vi "Get or Add Style Index.vi"(8 "error in":errorcluster, 10 "Format":string="dd/mm/yy hh:mm:ss.000", 11 "SpreadsheetDocument in":refnum<k24>) -> (0 "error out":errorcluster, 2 "Style Index":u32, 3 "SpreadsheetDocument out":refnum<k24>)   [LabVIEW 2021, in "Open Xml.lvlib"]
uses:
  Open Xml.lvlib
  D:/git/Open-Xml-LabVIEW/dll/DocumentFormat.OpenXml.dll
  dll/DocumentFormat.OpenXml.dll
  D:/git/Open-Xml-LabVIEW/dll/DocumentFormat.OpenXml.Framework.dll
  dll/DocumentFormat.OpenXml.Framework.dll
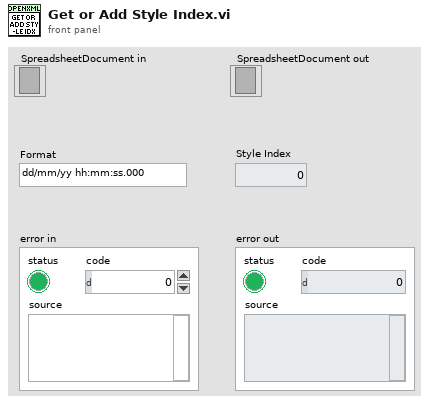
[diagram p1: front panel]
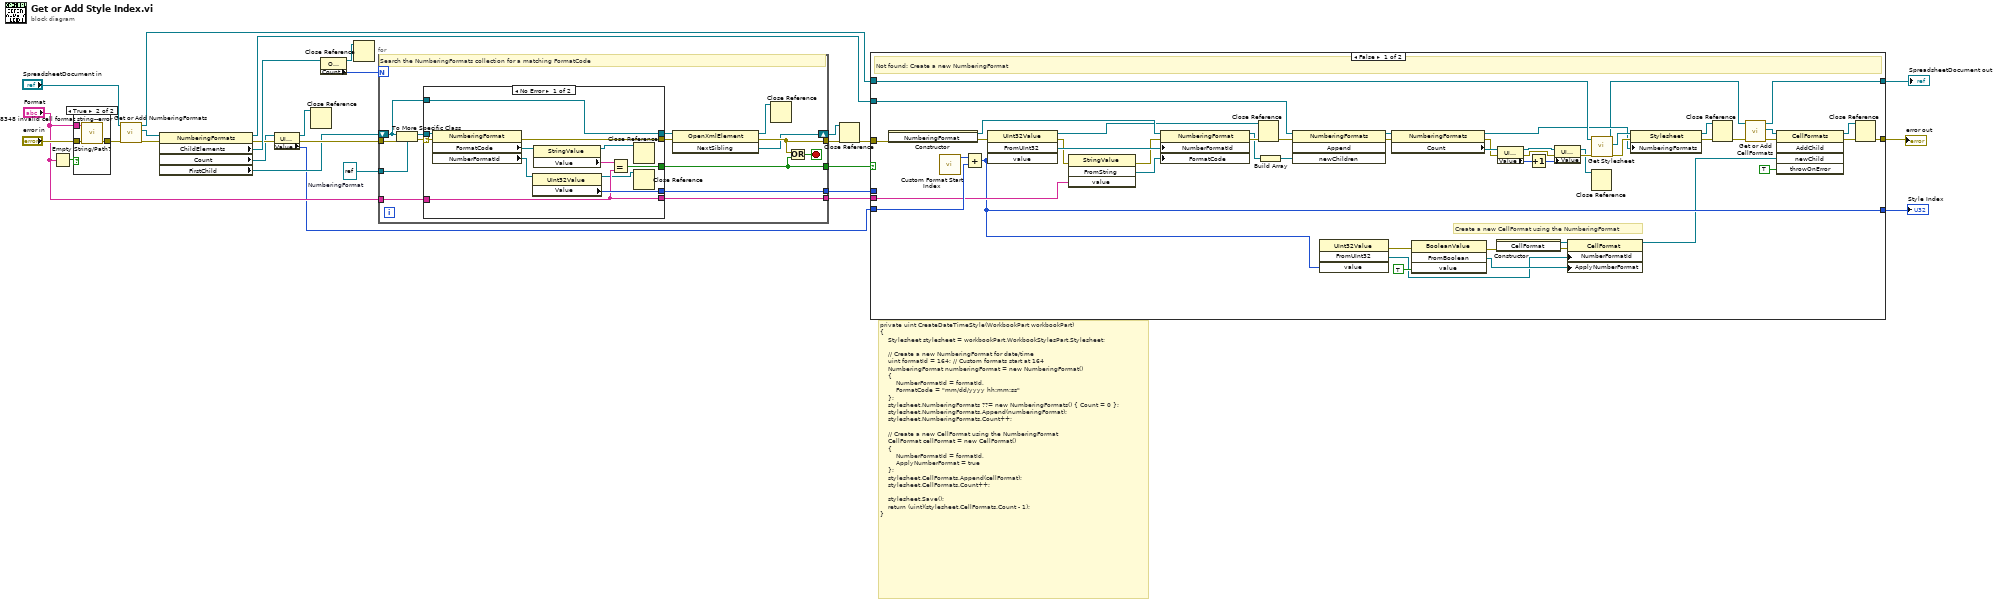
[diagram p0: block diagram]
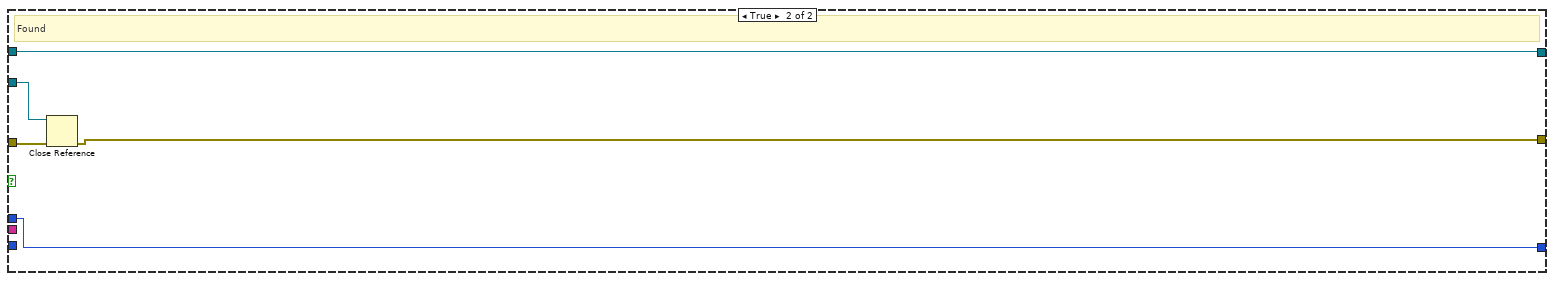
[diagram p2: hidden frame]
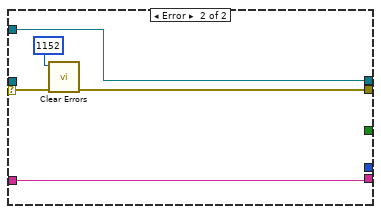
[diagram p4: hidden frame]
diagram:
  w22 = refnum<k24> refnum  # NumberingFormat
  # "private uint CreateDateTimeStyle(WorkbookPart workbookPart)\n{\n    Stylesheet stylesheet = workbookPart.WorkbookStylesPart.Stylesheet;\n\n    // Create a new NumberingFormat for date/time\n    uint formatId = 164; // Custom formats start at 164\n    NumberingFormat numberingFormat = new NumberingFormat()\n    {\n        NumberFormatId = formatId,\n        FormatCode = \"mm/dd/yyyy hh:mm:ss\"\n    };\n    stylesheet.NumberingFormats ??= new NumberingFormats() { Count = 0 };\n    stylesheet.NumberingFormats.Append(numberingFormat);\n    stylesheet.NumberingFormats.Count++;\n\n    // Create a new CellFormat using the NumberingFormat\n    CellFormat cellFormat = new CellFormat()\n    {\n        NumberFormatId = formatId,\n        ApplyNumberFormat = true\n    };\n    stylesheet.CellFormats.Append(cellFormat);\n    stylesheet.CellFormats.Count++;\n\n    stylesheet.Save();\n    return (uint)(stylesheet.CellFormats.Count - 1);\n}"
  n1 = Empty String/Path?(string/path="Format") -> (empty?=w19:bool)
  n2 = case shown="True" w19 {
    tunnel: "error in" -> [w29 w32]
    tunnel: [w29 w31] -> w20
    tunnel: "Format" -> [_ w30]
    frame False {
    }
    frame True {
      n3 = call "-8348 invalid cell format string--error.vi"("error in"=w32, "Argument"=w30) -> ("error out"=w31:errorcluster)  [unwired: 9 in]
    }
  }
  n4 = call "Get or Add NumberingFormats.vi"("error in"=w20, "SpreadsheetDoc in"="SpreadsheetDocument in") -> ("error out"=w27:errorcluster, "NumberingFormats"=w25:refnum<k24>, "SpreadsheetDoc out"=w7:refnum<k24>)  [unwired: 7 in]
  n5 = property class="NumberingFormats"(reference=w25, error in=w27) -> (reference out=w8:refnum<k24>, error out=w13:errorcluster, "ChildElements"=w24:refnum<k24>, "Count"=w11:refnum<k24>, "FirstChild"=w10:refnum<k24>)
  n6 = property class="UInt32Value"(reference=w11, error in=w13) -> (reference out=w3:refnum<k24>, error out=w12:errorcluster, "Value"=w9:u32)
  n7 = Close Reference(reference=w3) -> ()  [unwired: 1 in, 1 out]
  n8 = property class="OpenXmlElementList"(reference=w24) -> (reference out=w21:refnum<k24>, "Count"=w23:i32)  [unwired: 1 in, 1 out]
  n9 = Close Reference(reference=w21) -> ()  [unwired: 1 in, 1 out]
  n10 = for {
    N: w23 -> [_]
    tunnel: w12 -> [w46]
    tunnel: w22 -> [w47]
    shift-right: [w37] -> w1
    shift-left: w10 -> [w33]
    tunnel: [w39] -> w15
    tunnel: "Format" -> [w42]
    tunnel: [w40] -> w17
    tunnel: [w35] -> w16
    tunnel: [w34] -> w14
    stop <- w41 stop-if-true
    # "Search the NumberingFormats collection for a matching FormatCode"
    n11 = To More Specific Class(target class=w47, reference=w33, error in=w46) -> (specific class reference=w43:refnum<k24>, error out=w45:errorcluster)
    n12 = case shown="No Error" w45 {
      selector: w45 -> [w59 w64]
      tunnel: [w58 w63] -> w44
      tunnel: w43 -> [w57 _]
      tunnel: w42 -> [w51 w60]
      tunnel: [w54 _] -> w40
      tunnel: [w50 w61] -> w38
      tunnel: [w52 _] -> w35
      tunnel: [w51 w60] -> w34
      tunnel: w33 -> [w50 w61]
      frame No Error {
        n13 = property class="NumberingFormat"(reference=w57, error in=w59) -> (error out=w58:errorcluster, "FormatCode"=w56:refnum<k24>, "NumberFormatId"=w53:refnum<k24>)  [unwired: 1 out]
        n14 = property class="UInt32Value"(reference=w53) -> (reference out=w48:refnum<k24>, "Value"=w52:u32)  [unwired: 1 in, 1 out]
        n15 = property class="StringValue"(reference=w56) -> (reference out=w49:refnum<k24>, "Value"=w55:string)  [unwired: 1 in, 1 out]
        n16 = Equal?(x=w55, y=w51) -> (x = y?=w54:bool)
        n17 = Close Reference(reference=w49) -> ()  [unwired: 1 in, 1 out]
        n18 = Close Reference(reference=w48) -> ()  [unwired: 1 in, 1 out]
      }
      frame Error {
        n19 = call <vilib>:"Clear Errors.vi"("error in (no error)"=w64, "specific error code to clear (0: all)"=1152) -> ("error out"=w63:errorcluster)  [unwired: 4 in, 1 out]
      }
    }
    n20 = invoke class="OpenXmlElement" method="NextSibling"(reference=w38, error in=w44) -> (reference out=w36:refnum<k24>, error out=w39:errorcluster, "NextSibling"=w37:refnum<k24>)  [unwired: 1 in]
    n21 = Close Reference(reference=w36) -> ()  [unwired: 1 in, 1 out]
    n22 = Or(x=w39, y=w40) -> (x .or. y?=w41:bool)
  }
  n23 = Close Reference(reference=w1, error in (no error)=w15) -> (error out=w2:errorcluster)
  n24 = case shown="False" w17 {
    tunnel: w16 -> [_ w119]
    tunnel: w2 -> [w107 w116]
    tunnel: w14 -> [w93 _]
    tunnel: w9 -> [w106 _]
    tunnel: w8 -> [w105 w117]
    tunnel: w7 -> [w91 w118]
    tunnel: [w85 w115] -> w4
    tunnel: [w76 w118] -> w6
    tunnel: [w79 w119] -> w5
    frame False {
      # "Create a new CellFormat using the NumberingFormat"
      # "Not found: Create a new NumberingFormat"
      n25 = constructor class="NumberingFormat"(error in=w107) -> (reference out=w108:refnum<k24>, error out=w111:errorcluster)  [unwired: 2 in, 1 out]
      n26 = call "Custom Format Start Index.vi"() -> ("Start ID"=w109:u32)  [unwired: 11 in]
      n27 = Add(x=w109, y=w106) -> (x+y=w79:u32)
      n28 = invoke class="UInt32Value" method="FromUInt32"(error in=w111, "value"=w79) -> (reference out=w65:refnum<k24>, error out=w112:errorcluster, "FromUInt32"=w114:refnum<k24>)  [unwired: 2 in, 1 out]
      n29 = invoke class="StringValue" method="FromString"(error in=w112, "value"=w93) -> (error out=w113:errorcluster, "FromString"=w110:refnum<k24>)  [unwired: 2 in, 2 out]
      n30 = property class="NumberingFormat"(reference=w108, error in=w113, "NumberFormatId"=w114, "FormatCode"=w110) -> (reference out=w103:refnum<k24>, error out=w104:errorcluster)
      n31 = Close Reference(reference=w65, error in (no error)=w104) -> (error out=w66:errorcluster)
      n32 = Build Array(w103) -> (w102:refnum<k24>[])
      n33 = invoke class="NumberingFormats" method="Append"(reference=w105, error in=w66, "newChildren"=w102) -> (reference out=w100:refnum<k24>, error out=w101:errorcluster)  [unwired: 1 in, 2 out]
      n34 = invoke class="UInt32Value" method="FromUInt32"("value"=w79) -> (error out=w69:errorcluster, "FromUInt32"=w80:refnum<k24>)  [unwired: 3 in, 2 out]
      n35 = property class="NumberingFormats"(reference=w100, error in=w101) -> (reference out=w87:refnum<k24>, error out=w98:errorcluster, "Count"=w99:refnum<k24>)
      n36 = invoke class="BooleanValue" method="FromBoolean"(error in=w69, "value"=TRUE) -> (error out=w68:errorcluster, "FromBoolean"=w84:refnum<k24>)  [unwired: 2 in, 2 out]
      n37 = constructor class="CellFormat"(error in=w68) -> (reference out=w83:refnum<k24>, error out=w82:errorcluster)  [unwired: 2 in, 1 out]
      n38 = property class="UInt32Value"(reference=w99, error in=w98) -> (reference out=w94:refnum<k24>, error out=w95:errorcluster, "Value"=w97:u32)
      n39 = Increment(x=w97) -> (x+1=w96:u32)
      n40 = property class="UInt32Value"(reference=w94, error in=w95, "Value"=w96) -> (reference out=w89:refnum<k24>, error out=w90:errorcluster)
      n41 = property class="CellFormat"(reference=w83, error in=w82, "NumberFormatId"=w80, "ApplyNumberFormat"=w84) -> (reference out=w70:refnum<k24>)  [unwired: 1 out]
      n42 = Close Reference(reference=w89) -> ()  [unwired: 1 in, 1 out]
      n43 = call "Get Stylesheet.vi"("error in"=w90, "SpreadsheetDoc in"=w91) -> ("error out"=w88:errorcluster, "Stylesheet"=w92:refnum<k24>, "SpreadsheetDoc out"=w77:refnum<k24>)  [unwired: 7 in]
      n44 = property class="Stylesheet"(reference=w92, error in=w88, "NumberingFormats"=w87) -> (reference out=w72:refnum<k24>, error out=w86:errorcluster)
      n45 = Close Reference(reference=w72, error in (no error)=w86) -> (error out=w73:errorcluster)
      n46 = call "Get or Add CellFormats.vi"("error in"=w73, "SpreadsheetDoc in"=w77) -> ("error out"=w78:errorcluster, "CellFormats"=w74:refnum<k24>, "SpreadsheetDoc out"=w76:refnum<k24>)  [unwired: 7 in]
      n47 = invoke class="CellFormats" method="AddChild"(reference=w74, error in=w78, "newChild"=w70, "throwOnError"=TRUE) -> (reference out=w67:refnum<k24>, error out=w75:errorcluster)  [unwired: 1 in, 3 out]
      n48 = Close Reference(reference=w67, error in (no error)=w75) -> (error out=w85:errorcluster)
    }
    frame True {
      # "Found"
      n49 = Close Reference(reference=w117, error in (no error)=w116) -> (error out=w115:errorcluster)
    }
  }
  "SpreadsheetDocument out" <- w6
  "error out" <- w4
  "Style Index" <- w5
